vi "Dashboard_Cal_Globals.vi"() -> ()   [LabVIEW 2020]
panel:
  in  "Magazine_Firing_Throttle":dbl
  in  "Manual_Magazine_Power":dbl
  in  "Turret_Upper_Limit":dbl
  in  "Turret_Lower_Limit":dbl
  in  "Turret_Kd":dbl
  in  "Turret_Ki":dbl
  in  "Turret_Kp":dbl
  # "Add globals to the rest of the project."
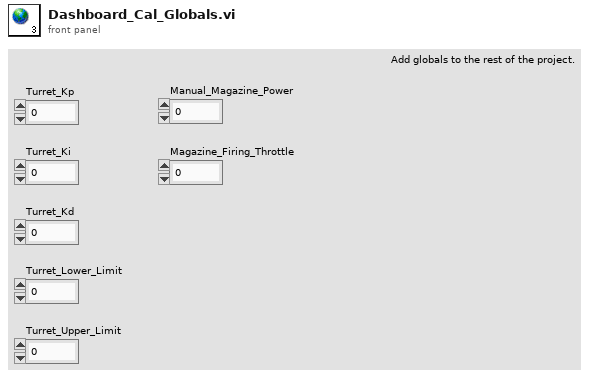
[diagram p1: front panel]
diagram:
